vi "各種價格.vi"(2 "Numeric":dbl) -> (5 "買空地":dbl, 6 "蓋房子":dbl, 7 "蓋旅館":dbl, 8 "1旅館費":dbl, 9 "空地費":dbl, 10 "1房子費":dbl)   [LabVIEW 2014]
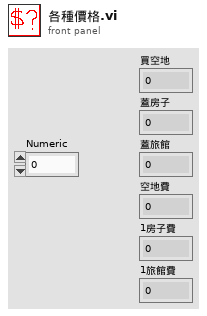
[diagram p1: front panel]
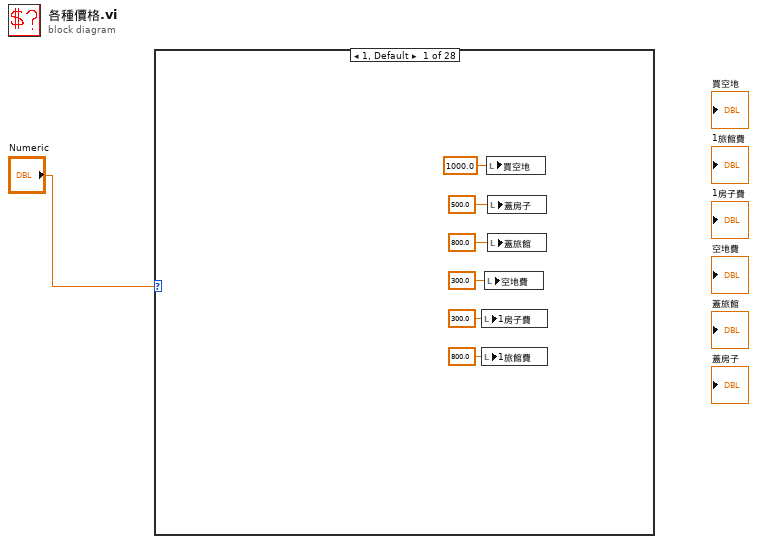
[diagram p0: block diagram]
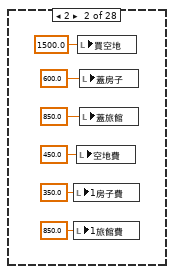
[diagram p2: hidden frame]
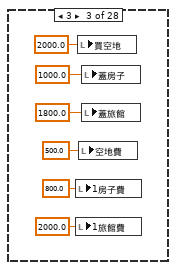
[diagram p3: hidden frame]
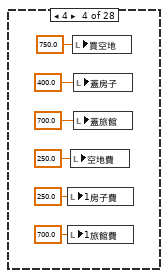
[diagram p4: hidden frame]
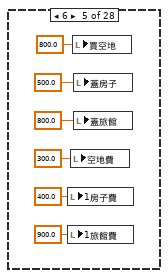
[diagram p5: hidden frame]
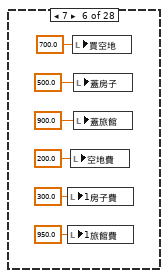
[diagram p6: hidden frame]
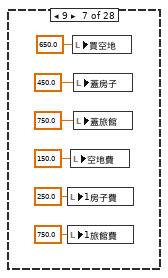
[diagram p7: hidden frame]
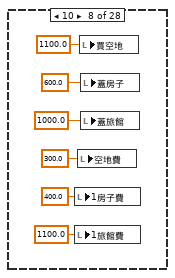
[diagram p8: hidden frame]
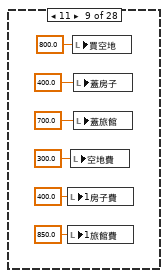
[diagram p9: hidden frame]
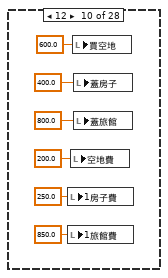
[diagram p10: hidden frame]
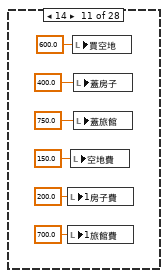
[diagram p11: hidden frame]
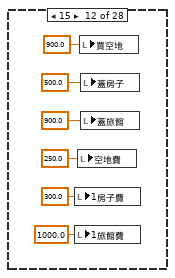
[diagram p12: hidden frame]
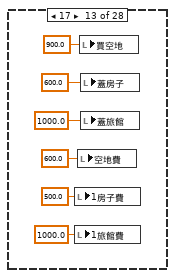
[diagram p13: hidden frame]
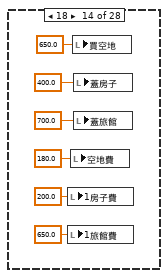
[diagram p14: hidden frame]
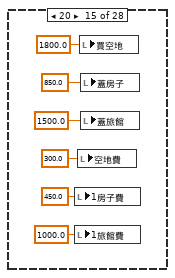
[diagram p15: hidden frame]
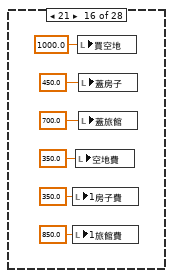
[diagram p16: hidden frame]
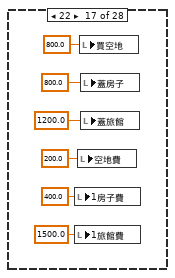
[diagram p17: hidden frame]
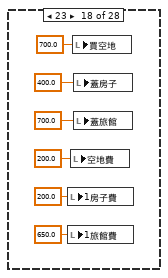
[diagram p18: hidden frame]
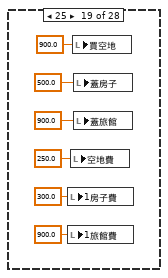
[diagram p19: hidden frame]
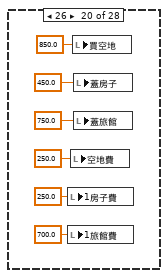
[diagram p20: hidden frame]
diagram:
  n1 = case shown="1, Default" "Numeric" {
    frame 1, Default {
      n2 = local write "1房子費"(300.0 ("蓋旅館")) -> ()
      n3 = local write "1旅館費"(800.0 ("蓋房子")) -> ()
      n4 = local write "空地費"(300.0 ("空地費")) -> ()
      n5 = local write "買空地"(1000.0 ("買空地")) -> ()
      n6 = local write "蓋房子"(500.0 ("1旅館費")) -> ()
      n7 = local write "蓋旅館"(800.0 ("1房子費")) -> ()
    }
    frame 2 {
      n8 = local write "1房子費"(350.0 ("蓋旅館")) -> ()
      n9 = local write "1旅館費"(850.0 ("蓋房子")) -> ()
      n10 = local write "空地費"(450.0 ("空地費")) -> ()
      n11 = local write "買空地"(1500.0 ("買空地")) -> ()
      n12 = local write "蓋房子"(600.0 ("1旅館費")) -> ()
      n13 = local write "蓋旅館"(850.0 ("1房子費")) -> ()
    }
    frame 3 {
      n14 = local write "1房子費"(800.0 ("蓋旅館")) -> ()
      n15 = local write "1旅館費"(2000.0 ("蓋房子")) -> ()
      n16 = local write "買空地"(2000.0 ("買空地")) -> ()
      n17 = local write "空地費"(500.0 ("空地費")) -> ()
      n18 = local write "蓋房子"(1000.0 ("1旅館費")) -> ()
      n19 = local write "蓋旅館"(1800.0 ("1房子費")) -> ()
    }
    frame 4 {
      n20 = local write "1房子費"(250.0 ("蓋旅館")) -> ()
      n21 = local write "1旅館費"(700.0 ("蓋房子")) -> ()
      n22 = local write "空地費"(250.0 ("空地費")) -> ()
      n23 = local write "買空地"(750.0 ("買空地")) -> ()
      n24 = local write "蓋房子"(400.0 ("1旅館費")) -> ()
      n25 = local write "蓋旅館"(700.0 ("1房子費")) -> ()
    }
    frame 6 {
      n26 = local write "1房子費"(400.0 ("蓋旅館")) -> ()
      n27 = local write "1旅館費"(900.0 ("蓋房子")) -> ()
      n28 = local write "空地費"(300.0 ("空地費")) -> ()
      n29 = local write "買空地"(800.0 ("買空地")) -> ()
      n30 = local write "蓋房子"(500.0 ("1旅館費")) -> ()
      n31 = local write "蓋旅館"(800.0 ("1房子費")) -> ()
    }
    frame 7 {
      n32 = local write "1房子費"(300.0 ("蓋旅館")) -> ()
      n33 = local write "1旅館費"(950.0 ("蓋房子")) -> ()
      n34 = local write "空地費"(200.0 ("空地費")) -> ()
      n35 = local write "買空地"(700.0 ("買空地")) -> ()
      n36 = local write "蓋房子"(500.0 ("1旅館費")) -> ()
      n37 = local write "蓋旅館"(900.0 ("1房子費")) -> ()
    }
    frame 9 {
      n38 = local write "1房子費"(250.0 ("蓋旅館")) -> ()
      n39 = local write "1旅館費"(750.0 ("蓋房子")) -> ()
      n40 = local write "空地費"(150.0 ("空地費")) -> ()
      n41 = local write "買空地"(650.0 ("買空地")) -> ()
      n42 = local write "蓋房子"(450.0 ("1旅館費")) -> ()
      n43 = local write "蓋旅館"(750.0 ("1房子費")) -> ()
    }
    frame 10 {
      n44 = local write "1房子費"(400.0 ("蓋旅館")) -> ()
      n45 = local write "1旅館費"(1100.0 ("蓋房子")) -> ()
      n46 = local write "空地費"(300.0 ("空地費")) -> ()
      n47 = local write "買空地"(1100.0 ("買空地")) -> ()
      n48 = local write "蓋房子"(600.0 ("1旅館費")) -> ()
      n49 = local write "蓋旅館"(1000.0 ("1房子費")) -> ()
    }
    frame 11 {
      n50 = local write "1房子費"(400.0 ("蓋旅館")) -> ()
      n51 = local write "1旅館費"(850.0 ("蓋房子")) -> ()
      n52 = local write "空地費"(300.0 ("空地費")) -> ()
      n53 = local write "買空地"(800.0 ("買空地")) -> ()
      n54 = local write "蓋房子"(400.0 ("1旅館費")) -> ()
      n55 = local write "蓋旅館"(700.0 ("1房子費")) -> ()
    }
    frame 12 {
      n56 = local write "1房子費"(250.0 ("蓋旅館")) -> ()
      n57 = local write "1旅館費"(850.0 ("蓋房子")) -> ()
      n58 = local write "空地費"(200.0 ("空地費")) -> ()
      n59 = local write "買空地"(600.0 ("買空地")) -> ()
      n60 = local write "蓋房子"(400.0 ("1旅館費")) -> ()
      n61 = local write "蓋旅館"(800.0 ("1房子費")) -> ()
    }
    frame 14 {
      n62 = local write "1房子費"(200.0 ("蓋旅館")) -> ()
      n63 = local write "1旅館費"(700.0 ("蓋房子")) -> ()
      n64 = local write "空地費"(150.0 ("空地費")) -> ()
      n65 = local write "買空地"(600.0 ("買空地")) -> ()
      n66 = local write "蓋房子"(400.0 ("1旅館費")) -> ()
      n67 = local write "蓋旅館"(750.0 ("1房子費")) -> ()
    }
    frame 15 {
      n68 = local write "1房子費"(300.0 ("蓋旅館")) -> ()
      n69 = local write "1旅館費"(1000.0 ("蓋房子")) -> ()
      n70 = local write "空地費"(250.0 ("空地費")) -> ()
      n71 = local write "買空地"(900.0 ("買空地")) -> ()
      n72 = local write "蓋房子"(500.0 ("1旅館費")) -> ()
      n73 = local write "蓋旅館"(900.0 ("1房子費")) -> ()
    }
    frame 17 {
      n74 = local write "1房子費"(500.0 ("蓋旅館")) -> ()
      n75 = local write "1旅館費"(1000.0 ("蓋房子")) -> ()
      n76 = local write "空地費"(600.0 ("空地費")) -> ()
      n77 = local write "買空地"(900.0 ("買空地")) -> ()
      n78 = local write "蓋房子"(600.0 ("1旅館費")) -> ()
      n79 = local write "蓋旅館"(1000.0 ("1房子費")) -> ()
    }
    frame 18 {
      n80 = local write "1房子費"(200.0 ("蓋旅館")) -> ()
      n81 = local write "1旅館費"(650.0 ("蓋房子")) -> ()
      n82 = local write "空地費"(180.0 ("空地費")) -> ()
      n83 = local write "買空地"(650.0 ("買空地")) -> ()
      n84 = local write "蓋房子"(400.0 ("1旅館費")) -> ()
      n85 = local write "蓋旅館"(700.0 ("1房子費")) -> ()
    }
    frame 20 {
      n86 = local write "1房子費"(450.0 ("蓋旅館")) -> ()
      n87 = local write "1旅館費"(1000.0 ("蓋房子")) -> ()
      n88 = local write "空地費"(300.0 ("空地費")) -> ()
      n89 = local write "買空地"(1800.0 ("買空地")) -> ()
      n90 = local write "蓋房子"(850.0 ("1旅館費")) -> ()
      n91 = local write "蓋旅館"(1500.0 ("1房子費")) -> ()
    }
    frame 21 {
      n92 = local write "1房子費"(350.0 ("蓋旅館")) -> ()
      n93 = local write "1旅館費"(850.0 ("蓋房子")) -> ()
      n94 = local write "空地費"(350.0 ("空地費")) -> ()
      n95 = local write "買空地"(1000.0 ("買空地")) -> ()
      n96 = local write "蓋房子"(450.0 ("1旅館費")) -> ()
      n97 = local write "蓋旅館"(700.0 ("1房子費")) -> ()
    }
    frame 22 {
      n98 = local write "1房子費"(400.0 ("蓋旅館")) -> ()
      n99 = local write "1旅館費"(1500.0 ("蓋房子")) -> ()
      n100 = local write "空地費"(200.0 ("空地費")) -> ()
      n101 = local write "買空地"(800.0 ("買空地")) -> ()
      n102 = local write "蓋房子"(800.0 ("1旅館費")) -> ()
      n103 = local write "蓋旅館"(1200.0 ("1房子費")) -> ()
    }
    frame 23 {
      n104 = local write "1房子費"(200.0 ("蓋旅館")) -> ()
      n105 = local write "1旅館費"(650.0 ("蓋房子")) -> ()
      n106 = local write "空地費"(200.0 ("空地費")) -> ()
      n107 = local write "買空地"(700.0 ("買空地")) -> ()
      n108 = local write "蓋房子"(400.0 ("1旅館費")) -> ()
      n109 = local write "蓋旅館"(700.0 ("1房子費")) -> ()
    }
    frame 25 {
      n110 = local write "1房子費"(300.0 ("蓋旅館")) -> ()
      n111 = local write "1旅館費"(900.0 ("蓋房子")) -> ()
      n112 = local write "空地費"(250.0 ("空地費")) -> ()
      n113 = local write "買空地"(900.0 ("買空地")) -> ()
      n114 = local write "蓋房子"(500.0 ("1旅館費")) -> ()
      n115 = local write "蓋旅館"(900.0 ("1房子費")) -> ()
    }
    frame 26 {
      n116 = local write "1房子費"(250.0 ("蓋旅館")) -> ()
      n117 = local write "1旅館費"(700.0 ("蓋房子")) -> ()
      n118 = local write "空地費"(250.0 ("空地費")) -> ()
      n119 = local write "買空地"(850.0 ("買空地")) -> ()
      n120 = local write "蓋房子"(450.0 ("1旅館費")) -> ()
      n121 = local write "蓋旅館"(750.0 ("1房子費")) -> ()
    }
    frame 27 {
      n122 = local write "1房子費"(200.0 ("蓋旅館")) -> ()
      n123 = local write "1旅館費"(600.0 ("蓋房子")) -> ()
      n124 = local write "空地費"(180.0 ("空地費")) -> ()
      n125 = local write "買空地"(650.0 ("買空地")) -> ()
      n126 = local write "蓋房子"(400.0 ("1旅館費")) -> ()
      n127 = local write "蓋旅館"(650.0 ("1房子費")) -> ()
    }
    frame 29 {
      n128 = local write "1房子費"(250.0 ("蓋旅館")) -> ()
      n129 = local write "1旅館費"(650.0 ("蓋房子")) -> ()
      n130 = local write "空地費"(250.0 ("空地費")) -> ()
      n131 = local write "買空地"(750.0 ("買空地")) -> ()
      n132 = local write "蓋房子"(450.0 ("1旅館費")) -> ()
      n133 = local write "蓋旅館"(700.0 ("1房子費")) -> ()
    }
    frame 30 {
      n134 = local write "1房子費"(300.0 ("蓋旅館")) -> ()
      n135 = local write "1旅館費"(750.0 ("蓋房子")) -> ()
      n136 = local write "空地費"(250.0 ("空地費")) -> ()
      n137 = local write "買空地"(700.0 ("買空地")) -> ()
      n138 = local write "蓋房子"(500.0 ("1旅館費")) -> ()
      n139 = local write "蓋旅館"(750.0 ("1房子費")) -> ()
    }
    frame 31 {
      n140 = local write "1房子費"(300.0 ("蓋旅館")) -> ()
      n141 = local write "1旅館費"(900.0 ("蓋房子")) -> ()
      n142 = local write "空地費"(350.0 ("空地費")) -> ()
      n143 = local write "買空地"(1200.0 ("買空地")) -> ()
      n144 = local write "蓋房子"(500.0 ("1旅館費")) -> ()
      n145 = local write "蓋旅館"(850.0 ("1房子費")) -> ()
    }
    frame 33 {
      n146 = local write "1房子費"(250.0 ("蓋旅館")) -> ()
      n147 = local write "1旅館費"(650.0 ("蓋房子")) -> ()
      n148 = local write "空地費"(200.0 ("空地費")) -> ()
      n149 = local write "買空地"(800.0 ("買空地")) -> ()
      n150 = local write "蓋房子"(450.0 ("1旅館費")) -> ()
      n151 = local write "蓋旅館"(750.0 ("1房子費")) -> ()
    }
    frame 34 {
      n152 = local write "1房子費"(300.0 ("蓋旅館")) -> ()
      n153 = local write "1旅館費"(800.0 ("蓋房子")) -> ()
      n154 = local write "空地費"(250.0 ("空地費")) -> ()
      n155 = local write "買空地"(900.0 ("買空地")) -> ()
      n156 = local write "蓋房子"(500.0 ("1旅館費")) -> ()
      n157 = local write "蓋旅館"(800.0 ("1房子費")) -> ()
    }
    frame 36 {
      n158 = local write "1房子費"(350.0 ("蓋旅館")) -> ()
      n159 = local write "1旅館費"(800.0 ("蓋房子")) -> ()
      n160 = local write "空地費"(400.0 ("空地費")) -> ()
      n161 = local write "買空地"(1300.0 ("買空地")) -> ()
      n162 = local write "蓋房子"(550.0 ("1旅館費")) -> ()
      n163 = local write "蓋旅館"(800.0 ("1房子費")) -> ()
    }
    frame 37 {
      n164 = local write "1房子費"(300.0 ("蓋旅館")) -> ()
      n165 = local write "1旅館費"(800.0 ("蓋房子")) -> ()
      n166 = local write "空地費"(300.0 ("空地費")) -> ()
      n167 = local write "買空地"(1000.0 ("買空地")) -> ()
      n168 = local write "蓋房子"(500.0 ("1旅館費")) -> ()
      n169 = local write "蓋旅館"(800.0 ("1房子費")) -> ()
    }
  }
